vi "Read Camera Status.vi"(8 "error in (no error)":errorcluster, 11 "CCDCamera in":refnum<class "CCDCamera.lvclass">) -> (0 "error out":errorcluster, 2 "Camera Status":T1, 3 "CCDCamera out":refnum<class "CCDCamera.lvclass">)   [LabVIEW 2018, in "CCDCamera.lvclass"]
uses:
  CCDCamera.lvclass
  CCDCamera.lvclass/CCDCamera.ctl
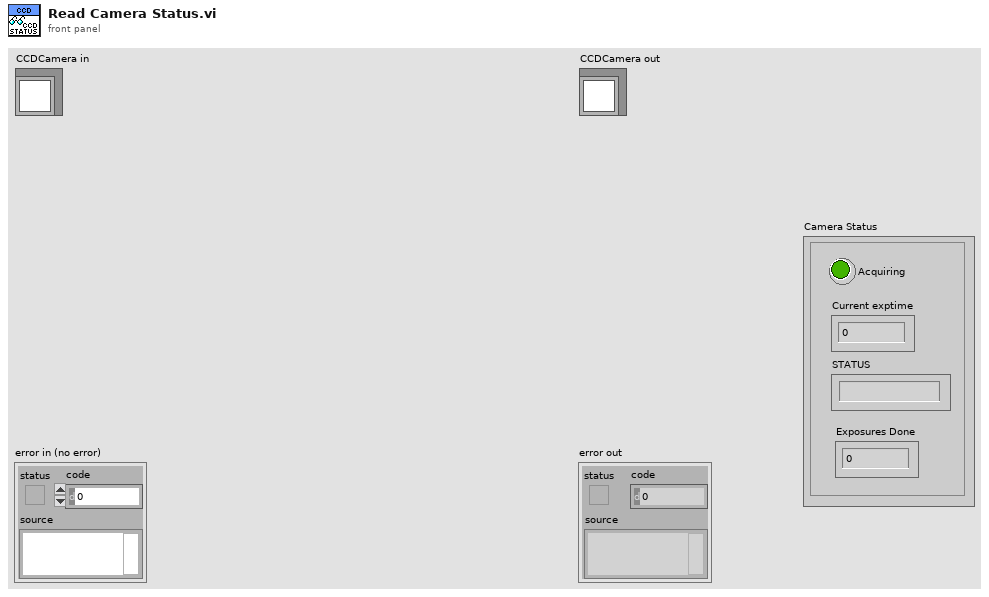
[diagram p1: front panel]
types:
  T1 = cluster{"Acquiring":bool, "Current exptime":sgl, "STATUS":string, "Exposures Done":u16}
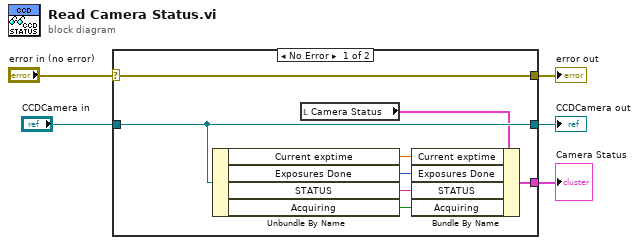
[diagram p0: block diagram]
diagram:
  n1 = case shown="No Error" "error in (no error)" {
    selector: "error in (no error)" -> [w12 w15]
    tunnel: [w12 w15] -> w5
    tunnel: [w13 w14] -> w4
    tunnel: "CCDCamera in" -> [w13 w14]
    tunnel: [w10 _] -> w1
    frame No Error {
      n2 = Unbundle By Name(w13) -> ("Current exptime"=w9:sgl, "Exposures Done"=w8:u16, "STATUS"=w7:string, "Acquiring"=w6:bool)
      n3 = local read "Camera Status"() -> (w11:T1)
      n4 = Bundle By Name(cluster=w11, "Current exptime"=w9, "Exposures Done"=w8, "STATUS"=w7, "Acquiring"=w6) -> (w10:T1)
    }
    frame Error {
    }
  }
  "error out" <- w5
  "CCDCamera out" <- w4
  "Camera Status" <- w1
